vi "SetUp.vi"(8 "error in (no error)":errorcluster, 11 "Prueba05 in":refnum<class "Prueba05.lvclass">) -> (0 "error out":errorcluster, 3 "Prueba05 out":refnum<class "Prueba05.lvclass">)   [LabVIEW 2019, in "Prueba05.lvclass"]
uses:
  Prueba05.lvclass
  Prueba05.lvclass/Prueba05.ctl
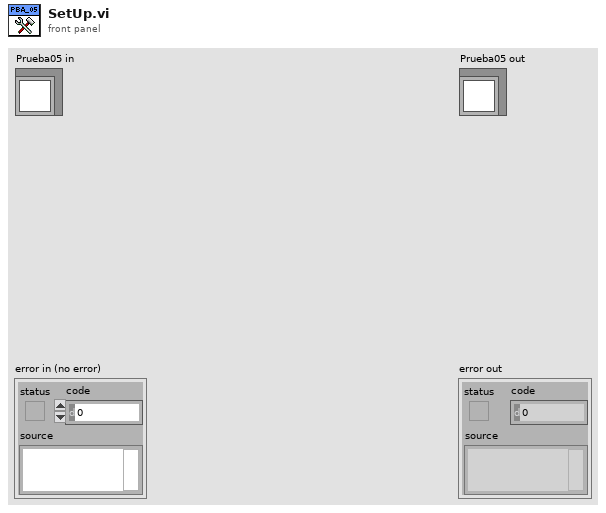
[diagram p1: front panel]
types:
  T1 = typedef "Prueba05.lvclass/BD.ctl" = cluster{"niv_presion_son_ref":dbl, "Incertidumbre":string[], "Tol +":string[], "Tol -":string[], "Frecuencias(Hz)":string[]}
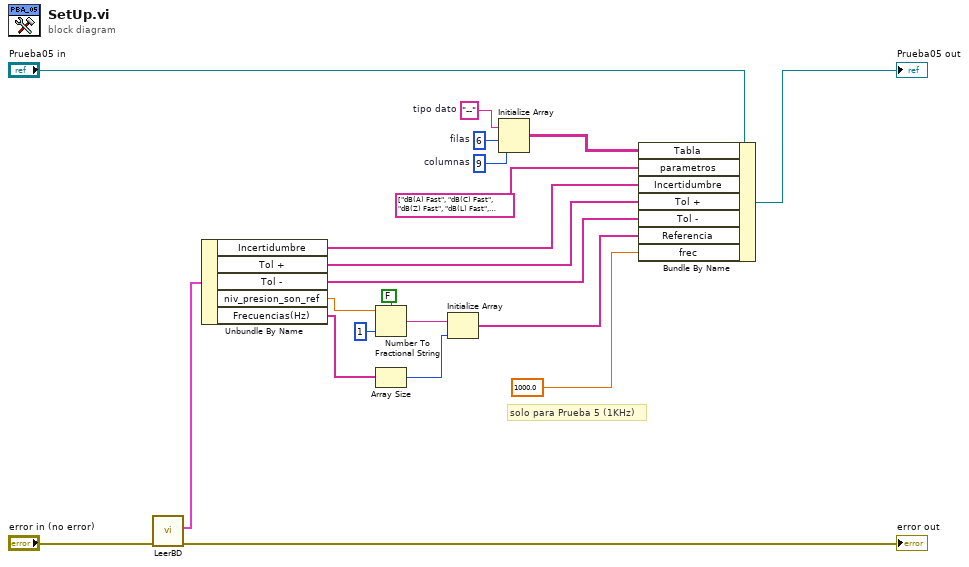
[diagram p0: block diagram]
diagram:
  w18 = 9  # columnas
  w19 = 6  # filas
  w17 = "--"  # tipo dato
  # "solo para Prueba 5 (1KHz)"
  n1 = call "LeerBD.vi"("error in (no error)"="error in (no error)") -> ("error out"=→"error out":errorcluster, "BD"=w11:T1)  [unwired: 8 in, 1 out]
  n2 = Unbundle By Name(w11) -> ("Incertidumbre"=w10:string[], "Tol +"=w9:string[], "Tol -"=w8:string[], "niv_presion_son_ref"=w7:dbl, "Frecuencias(Hz)"=w4:string[])
  n3 = Number To Fractional String(use system decimal point (T)=FALSE, number=w7, precision (6)=i16 1) -> (F-format string=w3:string)  [unwired: 1 in]
  n4 = Array Size(array=w4) -> (size(s)=w2:i32)
  n5 = Initialize Array(w3, w2) -> (w1:string[])
  n6 = Initialize Array(w17, w19, w18) -> (w15:string[][])
  n7 = Bundle By Name(cluster="Prueba05 in", "Tabla"=w15, "parametros"=string[] ["dB(A) Fast", "dB(C) Fast", "dB(Z) Fast", "dB(L) Fast", "dB(A) Slow", "Leq [dB(A)]"], "Incertidumbre"=w10, "Tol +"=w9, "Tol -"=w8, "Referencia"=w1, "frec"=1000.0 ("FrecAmpGEN.frec")) -> (→"Prueba05 out":refnum<class "Prueba05.lvclass">)
